vi "Open Selected VI.vi"(10 "Search Results":T3(array[cluster]), 11 "TreeControl in":refnum<vi>) -> ()   [LabVIEW 2019]
uses:
  Advanced Search.llb/Terminal Filter Output.ctl
  Advanced Search.llb/Terminals within Selection and GObject.ctl
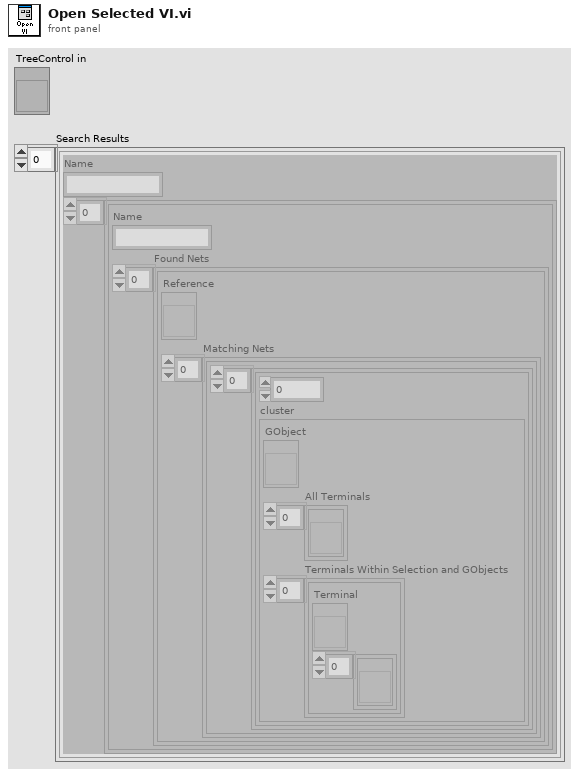
[diagram p1: front panel]
types:
  T1 = typedef "Terminal Filter Output.ctl" = cluster{"GObject":refnum<vi>, "All Terminals":refnum<vi>[], "Terminals Within Selection and GObjects":T2[]}
  T2 = typedef "Terminals within Selection and GObject.ctl" = cluster{"Terminal":refnum<vi>, "Attached GObjects":refnum<vi>[]}
  T3 = cluster{"Name":string, cluster{"Name":string, "Found Nets":cluster{"Reference":refnum<vi>, "Matching Nets":cluster{cluster{i32, "cluster":T1}[]}[]}[]}[]}[]
  T4 = enum32{"Invalid", "Standard", "Closed", "Hidden", "Minimized", "Maximized"}
  T5 = cluster{"Name":string, "Found Nets":cluster{"Reference":refnum<vi>, "Matching Nets":cluster{cluster{i32, "cluster":T1}[]}[]}[]}[]
  T6 = cluster{"Reference":refnum<vi>, "Matching Nets":cluster{cluster{i32, "cluster":T1}[]}[]}[]
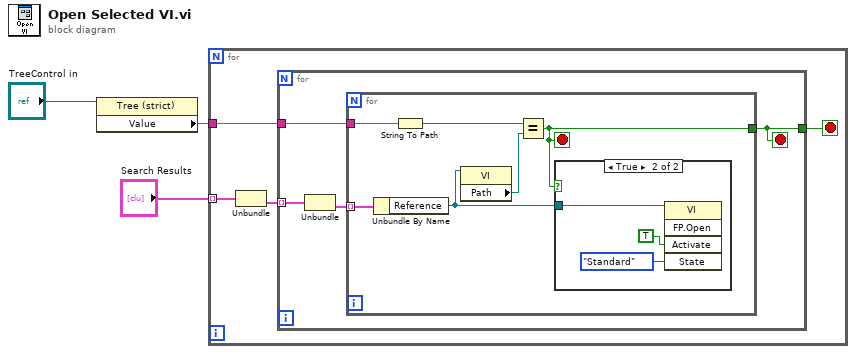
[diagram p0: block diagram]
diagram:
  n1 = property class="Tree (strict)"(reference="TreeControl in") -> ("Value"=w2:string)  [unwired: 1 in, 2 out]
  n2 = for {
    tunnel: "Search Results" -> [w7] mode=indexing
    tunnel: w2 -> [w5]
    stop <- w4 stop-if-true
    n3 = Unbundle(w7) -> (w6:T5)  [unwired: 1 out]
    n4 = for {
      tunnel: w6 -> [w11] mode=indexing
      tunnel: w5 -> [w9]
      tunnel: [w8] -> w4
      stop <- w8 stop-if-true
      n5 = Unbundle(w11) -> ("Found Nets"=w10:T6)  [unwired: 1 out]
      n6 = for {
        tunnel: w10 -> [w17] mode=indexing
        tunnel: w9 -> [w14]
        tunnel: [w13] -> w8
        stop <- w13 stop-if-true
        n7 = Unbundle By Name(w17) -> ("Reference"=w12:refnum<vi>)
        n8 = String To Path(string=w14) -> (path=w15:path)
        n9 = property class="VI"(reference=w12) -> ("Path"=w16:path)  [unwired: 1 in, 2 out]
        n10 = Equal?(x=w15, y=w16) -> (x = y?=w13:bool)
        n11 = case shown="True" w13 {
          tunnel: w12 -> [_ w18]
          frame False {
          }
          frame True {
            n12 = invoke class="VI" method="FP.Open"(reference=w18, "Activate"=TRUE ("Activate?"), "State"=T4."Standard") -> ()  [unwired: 2 in, 5 out]
          }
        }
      }
    }
  }
